vi "Stable_Capacitance_Check.vi"(7 "LowCapMode?":bool=TRUE, 8 "error in":errorcluster) -> (0 "error out":errorcluster, 2 "Capacitance (in pF)":dbl format="%.10g", 5 "Capacitance Stabilized":bool)   [LabVIEW 2020]
uses:
  Global 1.vi
  <vilib>/express/express arith-compare/Formula/XNode/ExpressFormulaBlockNode.xnode
panel:
  out "Outer While":i32
  out "Cap Sample 1":dbl format="%.10g"
  out "Cap Sample 2":dbl format="%.10g"
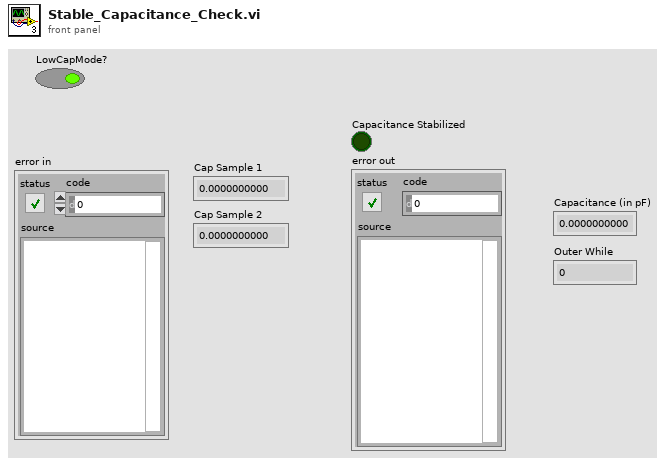
[diagram p1: front panel]
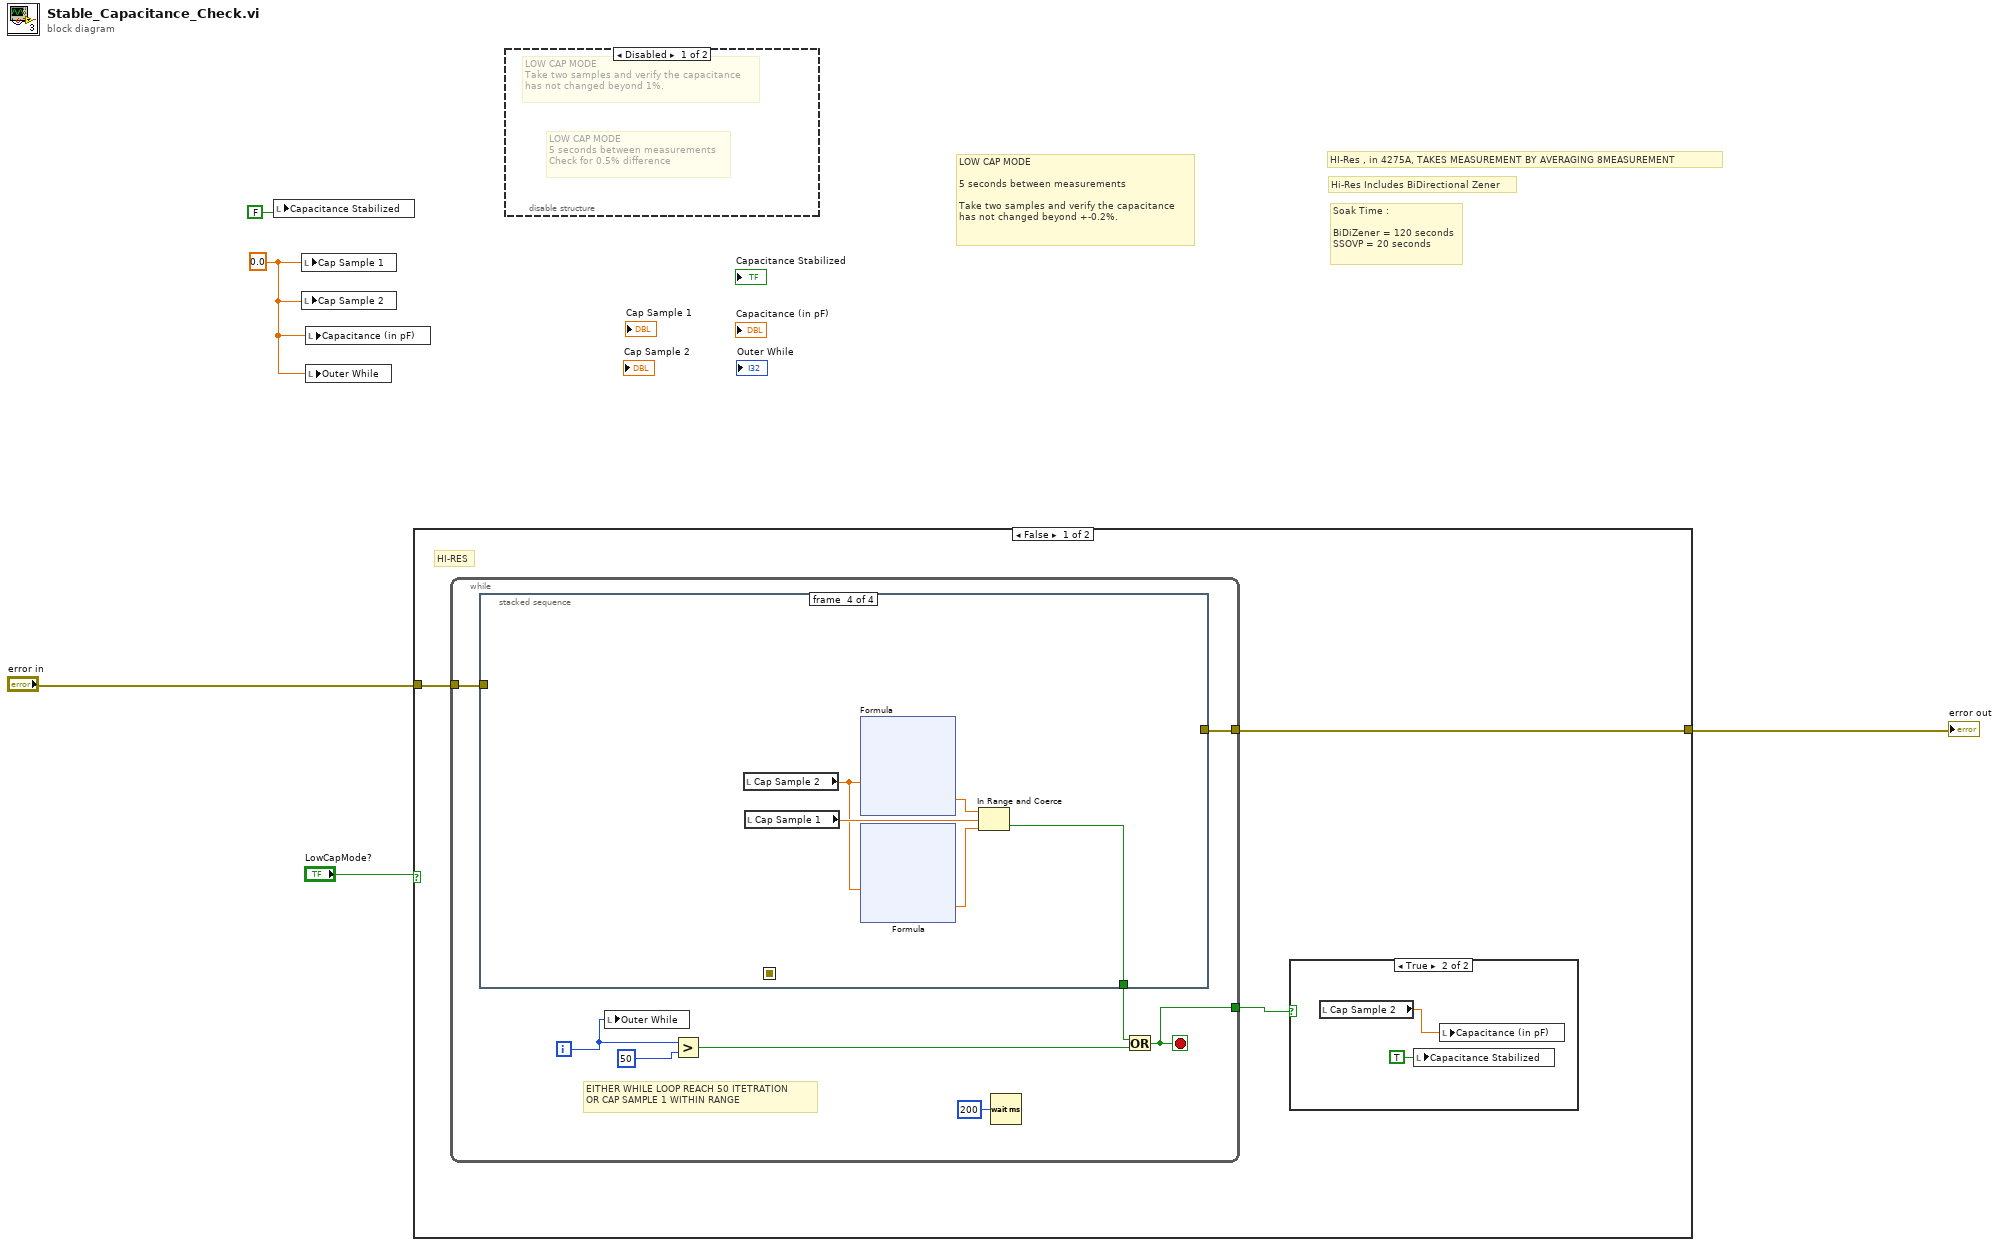
[diagram p0: block diagram]
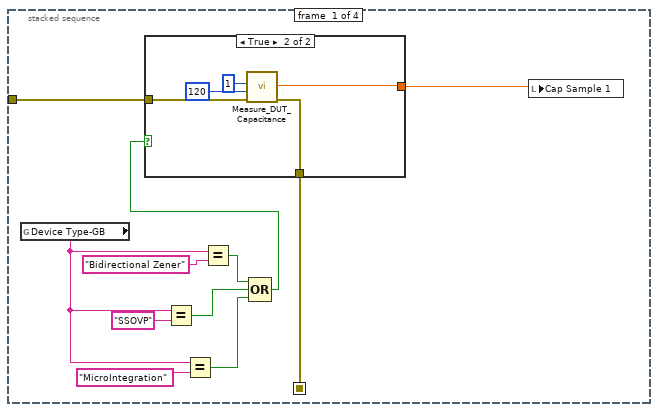
[diagram p4: hidden frame]
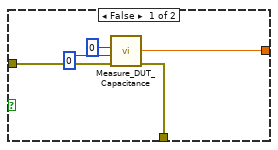
[diagram p5: hidden frame]
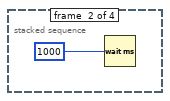
[diagram p6: hidden frame]
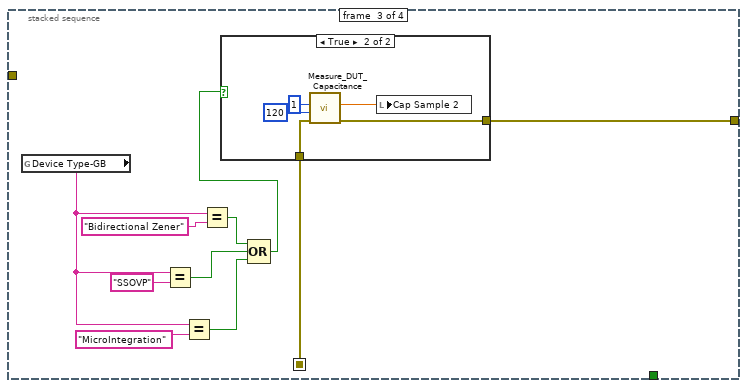
[diagram p7: hidden frame]
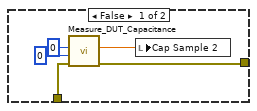
[diagram p8: hidden frame]
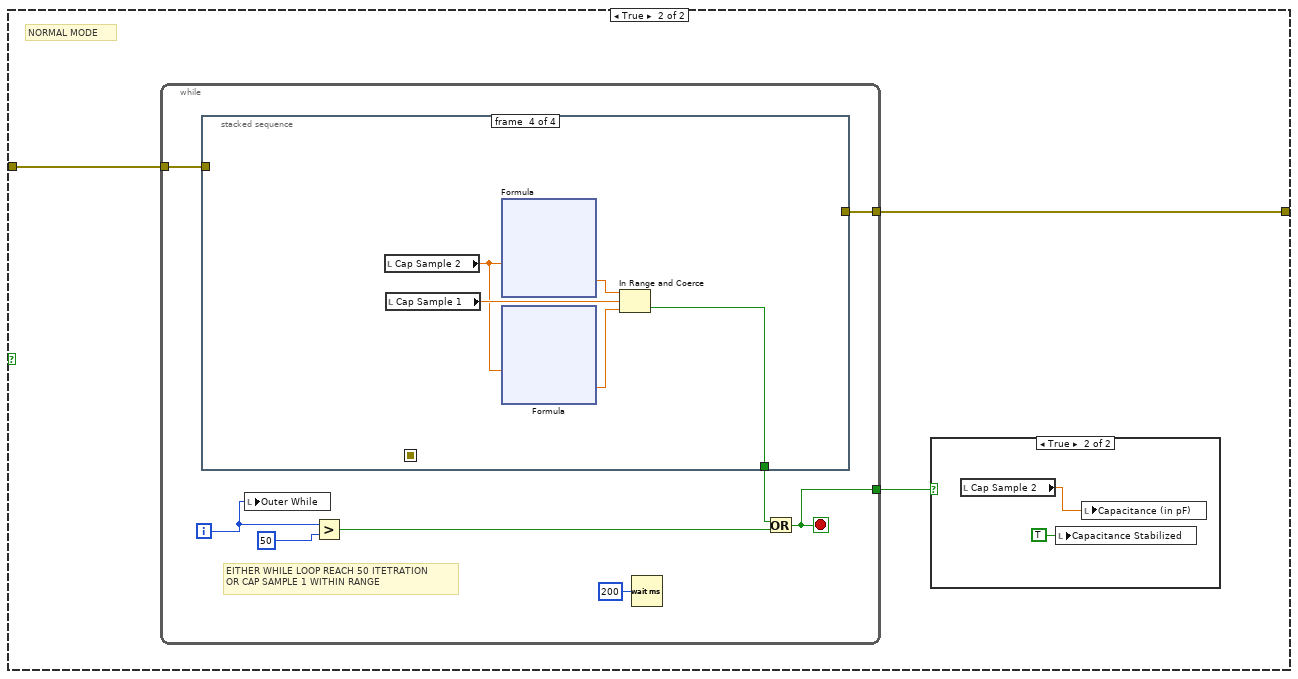
[diagram p9: hidden frame]
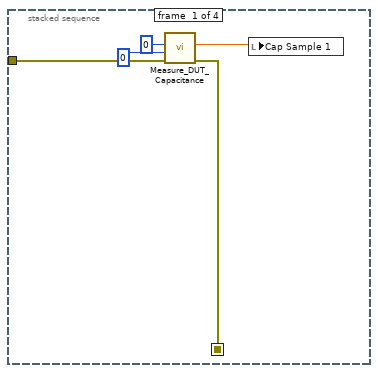
[diagram p11: hidden frame]
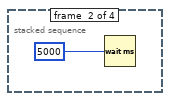
[diagram p12: hidden frame]
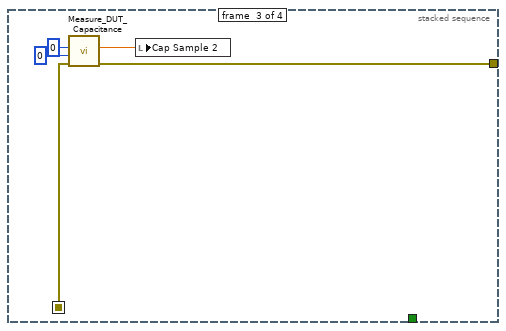
[diagram p13: hidden frame]
diagram:
  w1 = 0.0 ("Cap Sample 1")
  # "LOW CAP MODE\n\n5 seconds between measurements\n\nTake two samples and verify the capacitance\nhas not changed beyond +-0.2%."
  # "Soak Time :\n\nBiDiZener = 120 seconds\nSSOVP = 20 seconds"
  # "Hi-Res Includes BiDirectional Zener"
  # "HI-Res , in 4275A, TAKES MEASUREMENT BY AVERAGING 8MEASUREMENT"
  n1 = local write "Capacitance Stabilized"(FALSE ("Capacitance Stabilized")) -> ()
  n2 = local write "Cap Sample 1"(w1) -> ()
  n3 = local write "Cap Sample 2"(w1) -> ()
  n4 = local write "Capacitance (in pF)"(w1) -> ()
  n5 = local write "Outer While"(w1) -> ()
  n6 = case shown="False" "LowCapMode?" {
    tunnel: "error in" -> [w7 w84]
    tunnel: [w6 w83] -> w4
    frame False {
      # "HI-RES"
      n7 = while {
        tunnel: w7 -> [w18]
        tunnel: [w15] -> w6
        tunnel: [w14] -> w8
        i -> [w11]
        stop <- w14 stop-if-true
        # "EITHER WHILE LOOP REACH 50 ITETRATION\nOR CAP SAMPLE 1 WITHIN RANGE"
        n8 = stacked-sequence {
          seq-local: [w27 _ _ _] -> [_ _ w50 _]
          tunnel: w18 -> [w28 _ _ _]
          tunnel: [_ _ w49 _] -> w15
          tunnel: [_ _ _ w65] -> w13
          frame #0 {
            n9 = global read "Global 1.vi" "Device Type-GB"() -> (w20:string)
            n10 = Equal?(x=w20, y="SSOVP") -> (x = y?=w22:bool)
            n11 = Equal?(x=w20, y="MicroIntegration") -> (x = y?=w21:bool)
            n12 = Equal?(x=w20, y="Bidirectional Zener") -> (x = y?=w23:bool)
            n13 = Compound Arithmetic op=OR(w23, w22, w21) -> (w19:bool)
            n14 = case shown="True" w19 {
              tunnel: [w34 w35] -> w29
              tunnel: w28 -> [w33 w37]
              tunnel: [w32 w36] -> w27
              frame False {
                n15 = call "Measure_DUT_Capacitance.vi"("error in"=w33, "SoakTime"=u16 0, "AutoSoakFlag"=u16 0) -> ("error out"=w32:errorcluster, "Capacitance Data (in pF)"=w34:dbl)  [unwired: 5 in, 2 out]
              }
              frame True {
                n16 = call "Measure_DUT_Capacitance.vi"("error in"=w37, "SoakTime"=u16 120, "AutoSoakFlag"=u16 1) -> ("error out"=w36:errorcluster, "Capacitance Data (in pF)"=w35:dbl)  [unwired: 5 in, 2 out]
              }
            }
            n17 = local write "Cap Sample 1"(w29) -> ()
          }
          frame #1 {
            n18 = Wait (ms)(milliseconds to wait=u32 1000 ("t")) -> ()  [unwired: 1 out]
          }
          frame #2 {
            n19 = global read "Global 1.vi" "Device Type-GB"() -> (w45:string)
            n20 = Equal?(x=w45, y="SSOVP") -> (x = y?=w43:bool)
            n21 = Equal?(x=w45, y="MicroIntegration") -> (x = y?=w42:bool)
            n22 = Equal?(x=w45, y="Bidirectional Zener") -> (x = y?=w44:bool)
            n23 = Compound Arithmetic op=OR(w44, w43, w42) -> (w41:bool)
            n24 = case shown="True" w41 {
              tunnel: w50 -> [w52 w60]
              tunnel: [w51 w58] -> w49
              frame False {
                n25 = call "Measure_DUT_Capacitance.vi"("error in"=w52, "SoakTime"=u16 0, "AutoSoakFlag"=u16 0) -> ("error out"=w51:errorcluster, "Capacitance Data (in pF)"=w55:dbl)  [unwired: 5 in, 2 out]
                n26 = local write "Cap Sample 2"(w55) -> ()
              }
              frame True {
                n27 = call "Measure_DUT_Capacitance.vi"("error in"=w60, "SoakTime"=u16 120, "AutoSoakFlag"=u16 1) -> ("error out"=w58:errorcluster, "Capacitance Data (in pF)"=w59:dbl)  [unwired: 5 in, 2 out]
                n28 = local write "Cap Sample 2"(w59) -> ()
              }
            }
          }
          frame #3 {
            n29 = local read "Cap Sample 2"() -> (w61:dbl)
            n30 = local read "Cap Sample 1"() -> (w62:dbl)
            n31 = xnode "Formula"("X1"=w61) -> ("Result"=w64:dbl)  [unwired: 1 in, 1 out]
            n32 = xnode "Formula"("X1"=w61) -> ("Result"=w63:dbl)  [unwired: 1 in, 1 out]
            n33 = In Range and Coerce(upper limit=w64, x=w62, lower limit=w63) -> (In Range?=w65:bool)  [unwired: 1 out]
          }
        }
        n34 = local write "Outer While"(w11) -> ()
        n35 = Greater?(x=w11, y=50) -> (0:w16:bool)
        n36 = Wait (ms)(milliseconds to wait=u32 200) -> ()  [unwired: 1 out]
        n37 = Or(x=w13, y=w16) -> (x .or. y?=w14:bool)
      }
      n38 = case shown="True" w8 {
        frame False {
        }
        frame True {
          n39 = local read "Cap Sample 2"() -> (w9:dbl)
          n40 = local write "Capacitance Stabilized"(TRUE ("Capacitance Stabilized")) -> ()
          n41 = local write "Capacitance (in pF)"(w9) -> ()
        }
      }
    }
    frame True {
      # "NORMAL MODE"
      n42 = while {
        tunnel: w84 -> [w94]
        tunnel: [w91] -> w83
        tunnel: [w90] -> w82
        i -> [w87]
        stop <- w90 stop-if-true
        # "EITHER WHILE LOOP REACH 50 ITETRATION\nOR CAP SAMPLE 1 WITHIN RANGE"
        n43 = stacked-sequence {
          seq-local: [w97 _ _ _] -> [_ _ w105 _]
          tunnel: w94 -> [w98 _ _ _]
          tunnel: [_ _ w103 _] -> w91
          tunnel: [_ _ _ w110] -> w89
          frame #0 {
            n44 = call "Measure_DUT_Capacitance.vi"("error in"=w98, "SoakTime"=u16 0, "AutoSoakFlag"=u16 0) -> ("error out"=w97:errorcluster, "Capacitance Data (in pF)"=w99:dbl)  [unwired: 5 in, 2 out]
            n45 = local write "Cap Sample 1"(w99) -> ()
          }
          frame #1 {
            n46 = Wait (ms)(milliseconds to wait=u32 5000 ("t")) -> ()  [unwired: 1 out]
          }
          frame #2 {
            n47 = call "Measure_DUT_Capacitance.vi"("error in"=w105, "SoakTime"=u16 0, "AutoSoakFlag"=u16 0) -> ("error out"=w103:errorcluster, "Capacitance Data (in pF)"=w104:dbl)  [unwired: 5 in, 2 out]
            n48 = local write "Cap Sample 2"(w104) -> ()
          }
          frame #3 {
            n49 = local read "Cap Sample 2"() -> (w106:dbl)
            n50 = local read "Cap Sample 1"() -> (w107:dbl)
            n51 = xnode "Formula"("X1"=w106) -> ("Result"=w109:dbl)  [unwired: 1 in, 1 out]
            n52 = xnode "Formula"("X1"=w106) -> ("Result"=w108:dbl)  [unwired: 1 in, 1 out]
            n53 = In Range and Coerce(upper limit=w109, x=w107, lower limit=w108) -> (In Range?=w110:bool)  [unwired: 1 out]
          }
        }
        n54 = local write "Outer While"(w87) -> ()
        n55 = Greater?(x=w87, y=50) -> (0:w92:bool)
        n56 = Wait (ms)(milliseconds to wait=u32 200) -> ()  [unwired: 1 out]
        n57 = Or(x=w89, y=w92) -> (x .or. y?=w90:bool)
      }
      n58 = case shown="True" w82 {
        frame False {
        }
        frame True {
          n59 = local read "Cap Sample 2"() -> (w85:dbl)
          n60 = local write "Capacitance Stabilized"(TRUE ("Capacitance Stabilized")) -> ()
          n61 = local write "Capacitance (in pF)"(w85) -> ()
        }
      }
    }
  }
  "error out" <- w4
  n62 = disable-structure shown="Disabled" {
    frame Disabled {
      # "LOW CAP MODE\n5 seconds between measurements\nCheck for 0.5% difference"
      # "LOW CAP MODE\nTake two samples and verify the capacitance\nhas not changed beyond 1%."
    }
    frame Enabled {
    }
  }
